vi "XY to Waveform.vi"   [LabVIEW 2019, in "xy_utilities.lvlib"]
doc: "Convert <b>XY-data</b> to <b>Waveform</b>.\n\nWire data to the data input to determine the polymorphic instance to use or manually select the instance."
uses:
  xy_utilities.lvlib
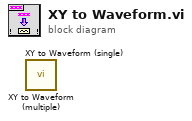
[diagram p0: block diagram]
diagram:
  n1 = call "XY to Waveform (multiple).vi"() -> ()  [unwired: 9 in, 3 out]
  n2 = call "XY to Waveform (single).vi"() -> ()  [unwired: 9 in, 3 out]
